vi "Factorial.vi"() -> ()   [LabVIEW 2018]
panel:
  in  "Numeric":dbl
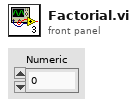
[diagram p1: front panel]
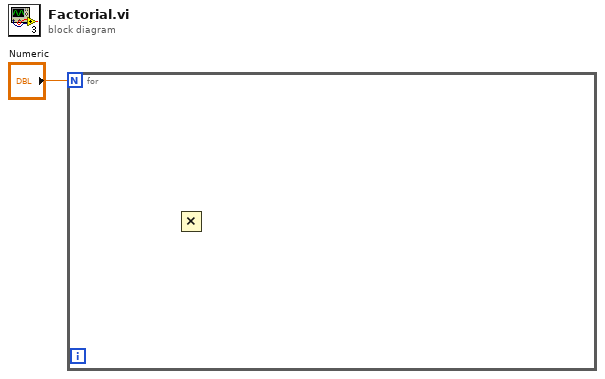
[diagram p0: block diagram]
diagram:
  n1 = for {
    N: "Numeric" -> [_]
    n2 = Multiply() -> ()  [unwired: 2 in, 1 out]
  }
